vi "Wait For Good Link.vi"(0 "Refnum in":refnum<k20>, 5 "Port":T1 items=["Port 0", "Port 1", "Port 2", "Port 3"], 11 "error in":errorcluster) -> (4 "Refnum out":refnum<k20>, 6 "Port Debug Info":T2, 15 "error out":errorcluster)   [LabVIEW 2016, in "Aurora Stream (NI 6592R) (Host).lvlib"]
doc: "Waits until the link is up and running and without error.\nAfter this VI completes, the Aurora core should be fully up and running and ready to transmit and receive data.\n\n<B>Input Parameters</B>\n\n<B>Refnum in</B> Receives a reference to the FPGA from the previous VI.\n\n<B>Port</B> Specifies the port on which to check if the UserClk is running.\n\n<B>error in</B> describes error conditions that occur before this node runs. This input provides standard error in functionality.\n\n<B>Output Parameters</B>\n\n<B>Refnum out</B> passes a reference to the FPGA to the next VI.\n\n<B>Port Debug Info</B> contains debug information related to the specified Port's link status.\n\n<B>Port Debug Info.Hard Error</B> indicates whether a hard error has occurred within the Aurora core.\n\n<B>Port Debug Info.Soft Error</B> indicates whether a soft error has occurred within the Aurora core.\n\n<B>Port Debug Info.Lane Up</B> indicates whether the lanes on the specified Port are up. This contains a bitwise OR of the status of the four lanes coming from the Aurora core.\n\n<B>Port Debug Info.Channel Up</B> indicates whether the channel is up.\n\n<B>Port Debug Info.Sys Reset</B> indicates whether the Aurora core is in System reset.\n\n<B>error out</B> contains error information. This output provides standard error out functionality."
uses:
  Aurora Stream (NI 6592R) (Host).lvlib
  Port.ctl
  Base Bitfile Reference.ctl
  <vilib>/Utility/error.llb/Error Cluster From Error Code.vi
  <vilib>/rvi/errors/niLvFpgaAdjustHostInterfaceError.vi
  <vilib>/rvi/interface/nirviReadWriteControl/nirviReadWriteControl.xnode
  <vilib>/rvi/interface/Simulation/niFpgaSimulationCallBeginRW.vi
  NiFpgaLv.dll
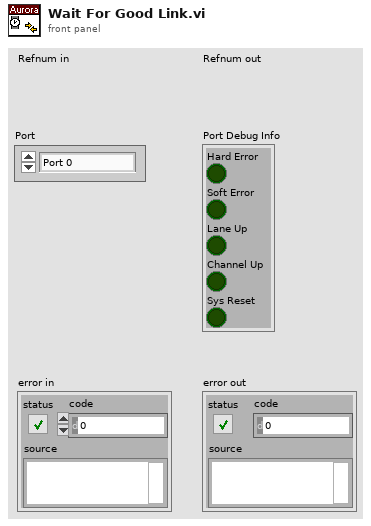
[diagram p1: front panel]
types:
  T1 = typedef "Aurora Stream (NI 6592R) (Host).lvlib/Port.ctl" = i32
  T2 = cluster{"Hard Error":bool, "Soft Error":bool, "Lane Up":bool, "Channel Up":bool, "Sys Reset":bool}
  T3 = typedef "Aurora Stream (NI 6592R) (Host).lvlib/Base Bitfile Reference.ctl" = refnum<k20>
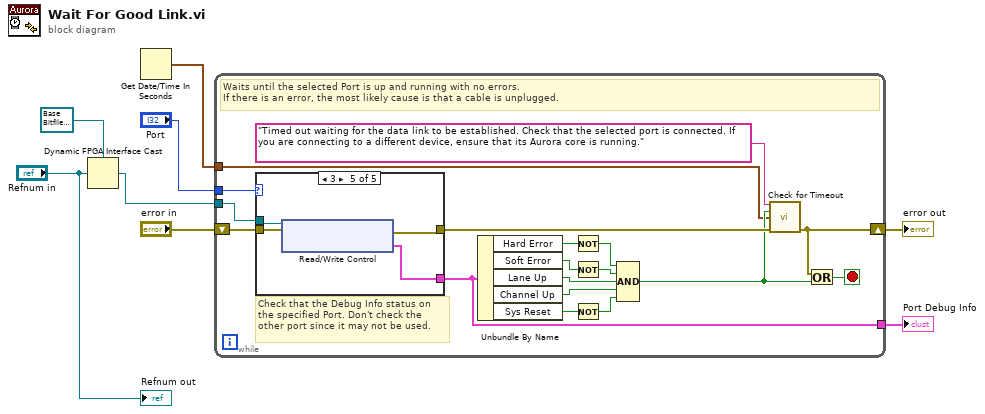
[diagram p0: block diagram]
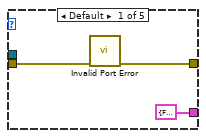
[diagram p2: hidden frame]
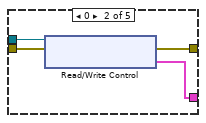
[diagram p3: hidden frame]
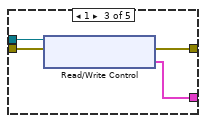
[diagram p4: hidden frame]
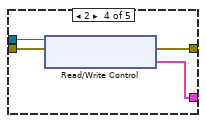
[diagram p5: hidden frame]
diagram:
  n1 = Dynamic FPGA Interface Cast(Session In=T3 refnum ("Aurora Sample Project"), Type="Refnum in") -> (Session Out=w2:T3)
  n2 = Get Date/Time In Seconds() -> (seconds since 1Jan1904=w8:timestamp)
  n3 = while {
    shift-right: [w13] -> w4
    shift-left: "error in" -> [w24]
    tunnel: w8 -> [w9]
    tunnel: [w23] -> w5
    tunnel: "Port" -> [w14]
    tunnel: w2 -> [w25]
    stop <- w26 stop-if-true
    # "Check that the Debug Info status on\nthe specified Port. Don't check the \nother port since it may not be used."
    # "Waits until the selected Port is up and running with no errors.\nIf there is an error, the most likely cause is that a cable is unplugged."
    n4 = case shown="3" w14 {
      tunnel: w25 -> [_ w33 w36 w41 w44]
      tunnel: w24 -> [w28 w32 w37 w40 w45]
      tunnel: [w27 w31 w35 w39 w43] -> w12
      tunnel: [T2 {"Hard Error"=FALSE, "Soft Error"=FALSE, "Lane Up"=FALSE, "Channel Up"=FALSE, "Sys Reset"=FALSE} ("Port 0 Debug Info") w30 w34 w38 w42] -> w23
      frame Default {
        n5 = call "Invalid Port Error.vi"("error in"=w28) -> ("error out"=w27:errorcluster)  [unwired: 14 in]
      }
      frame 0 {
        n6 = xnode "Read/Write Control"("FPGA VI Reference In"=w33, "error in"=w32) -> ("error out"=w31:errorcluster, "Port 0 Debug Info"=w30:T2)  [unwired: 1 out]
      }
      frame 1 {
        n7 = xnode "Read/Write Control"("FPGA VI Reference In"=w36, "error in"=w37) -> ("error out"=w35:errorcluster, "Port 1 Debug Info"=w34:T2)  [unwired: 1 out]
      }
      frame 2 {
        n8 = xnode "Read/Write Control"("FPGA VI Reference In"=w41, "error in"=w40) -> ("error out"=w39:errorcluster, "Port 2 Debug Info"=w38:T2)  [unwired: 1 out]
      }
      frame 3 {
        n9 = xnode "Read/Write Control"("FPGA VI Reference In"=w44, "error in"=w45) -> ("error out"=w43:errorcluster, "Port 3 Debug Info"=w42:T2)  [unwired: 1 out]
      }
    }
    n10 = Unbundle By Name(w23) -> ("Hard Error"=w22:bool, "Soft Error"=w21:bool, "Lane Up"=w20:bool, "Channel Up"=w19:bool, "Sys Reset"=w18:bool)
    n11 = Not(x=w22) -> (.not. x?=w16:bool)
    n12 = Not(x=w21) -> (.not. x?=w17:bool)
    n13 = Not(x=w18) -> (.not. x?=w15:bool)
    n14 = Compound Arithmetic op=AND(w16, w17, w20, w19, w15) -> (w10:bool)
    n15 = call "Check for Timeout.vi"("Error Message"="Timed out waiting for the data link to be established. Check that the selected port is connected. If you are connecting to a different device, ensure that its Aurora core is running." ("error message (\"\")"), "Complete?"=w10, "Start Time"=w9, "error in"=w12) -> ("error out"=w13:errorcluster)  [unwired: 11 in]
    n16 = Or(x=w13, y=w10) -> (x .or. y?=w26:bool)
  }
  "error out" <- w4
  "Port Debug Info" <- w5
  "Refnum out" <- "Refnum in"
